vi "Timing.vi"(8 "error in":errorcluster, 9 "Stabilization\nInterval":dbl, 10 "Timing":refnum<queue>, 11 "UI":refnum<queue>) -> (0 "error out":errorcluster)   [LabVIEW 2013]
uses:
  MeasurementControl Message Queue Folder/Message Cluster.ctl
  MeasurementControl Message Queue Folder/Enqueue Message (Single).vi
  MeasurementControl Message Queue Folder/MeasurementControl Message Queue.lvlib
panel:
  out "Naked Sphere Time Left":dbl
  out "Insulated Sphere Time Left":dbl
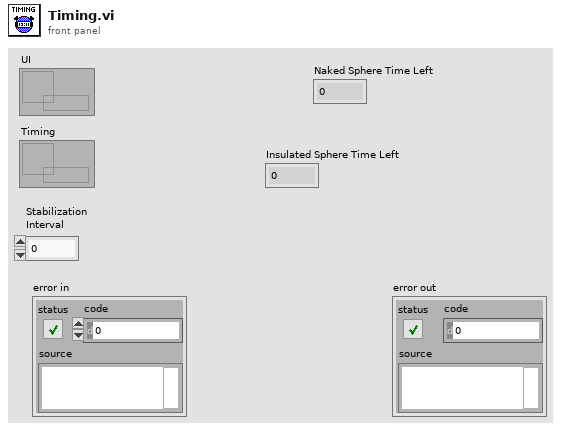
[diagram p1: front panel]
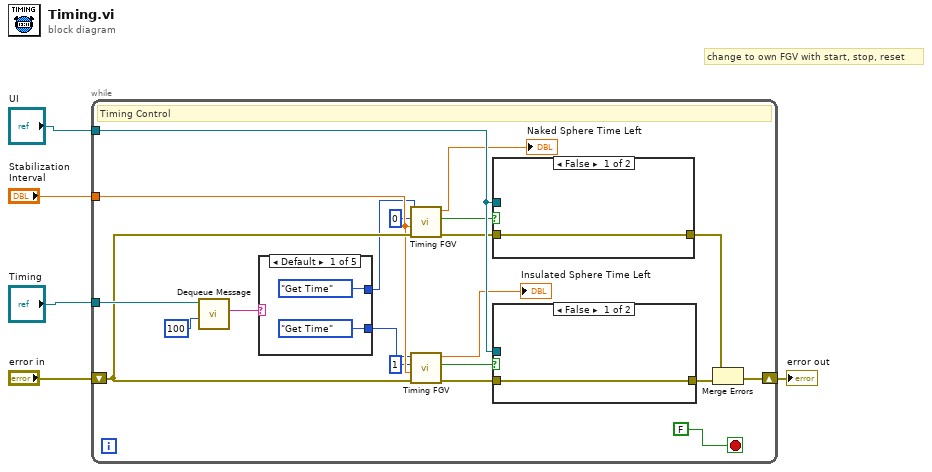
[diagram p0: block diagram]
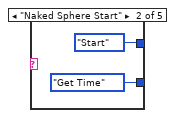
[diagram p2: hidden frame]
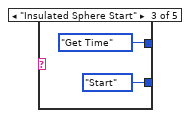
[diagram p3: hidden frame]
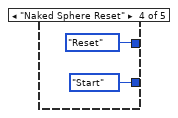
[diagram p4: hidden frame]
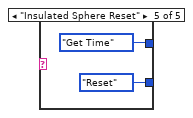
[diagram p5: hidden frame]
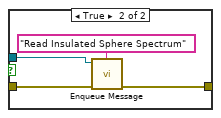
[diagram p6: hidden frame]
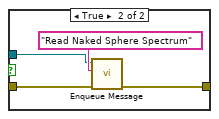
[diagram p7: hidden frame]
diagram:
  # "change to own FGV with start, stop, reset"
  n1 = while {
    shift-right: [w22] -> w1
    shift-left: "error in" -> [w18]
    tunnel: "Timing" -> [w24]
    tunnel: "Stabilization\nInterval" -> [w15]
    tunnel: "UI" -> [w20]
    stop <- FALSE stop-if-true
    # "Timing Control"
    n2 = call "Dequeue Message.vi"("timeout in ms (-1)"=100, "Message Queue"=w24) -> ("Message"=w8:string)  [unwired: 6 in, 3 out]
    n3 = case shown="Default" w8 {
      tunnel: [enum16{"Start", "Stop", "Reset", "Get Time"}."Get Time" ("Method (Get Time)") enum16{"Start", "Stop", "Reset", "Get Time"}."Start" ("Method (Get Time)") enum16{"Start", "Stop", "Reset", "Get Time"}."Get Time" ("Method (Get Time)") enum16{"Start", "Stop", "Reset", "Get Time"}."Reset" ("Method (Get Time)") enum16{"Start", "Stop", "Reset", "Get Time"}."Get Time" ("Method (Get Time)")] -> w7
      tunnel: [enum16{"Start", "Stop", "Reset", "Get Time"}."Get Time" ("Method (Get Time)") enum16{"Start", "Stop", "Reset", "Get Time"}."Get Time" ("Method (Get Time)") enum16{"Start", "Stop", "Reset", "Get Time"}."Start" ("Method (Get Time)") enum16{"Start", "Stop", "Reset", "Get Time"}."Start" ("Method (Get Time)") enum16{"Start", "Stop", "Reset", "Get Time"}."Reset" ("Method (Get Time)")] -> w6
      frame Default {
      }
      frame "Naked Sphere Start" {
      }
      frame "Insulated Sphere Start" {
      }
      frame "Naked Sphere Reset" {
      }
      frame "Insulated Sphere Reset" {
      }
    }
    n4 = call "Timing FGV.vi"("error in (no error)"=w18, "Target time (s)"=w15, "Index"=0, "Method (Get Time)"=w7) -> ("error out"=w10:errorcluster, "Done"=w17:bool, "Time Remaining(s)"=→"Naked Sphere Time Left":dbl)  [unwired: 5 in]
    n5 = call "Timing FGV.vi"("error in (no error)"=w18, "Target time (s)"=w15, "Index"=1, "Method (Get Time)"=w6) -> ("error out"=w9:errorcluster, "Done"=w16:bool, "Time Remaining(s)"=→"Insulated Sphere Time Left":dbl)  [unwired: 5 in]
    n6 = case shown="False" w17 {
      tunnel: [w41 w45] -> w23
      tunnel: w20 -> [_ w43]
      tunnel: w10 -> [w41 w42]
      frame False {
      }
      frame True {
        n7 = call-poly "Enqueue Message.vi"("error in (no error)"=w42, "Message"="Read Naked Sphere Spectrum", "Message Queue"=w43) -> ("error out"=w45:errorcluster)  [unwired: 7 in, 1 out]
      }
    }
    n8 = case shown="False" w16 {
      tunnel: [w36 w40] -> w21
      tunnel: w20 -> [_ w38]
      tunnel: w9 -> [w36 w37]
      frame False {
      }
      frame True {
        n9 = call-poly "Enqueue Message.vi"("error in (no error)"=w37, "Message"="Read Insulated Sphere Spectrum", "Message Queue"=w38) -> ("error out"=w40:errorcluster)  [unwired: 7 in, 1 out]
      }
    }
    n10 = Merge Errors(w23, w21) -> (w22:errorcluster)
  }
  "error out" <- w1
